vi "Status.Builder.New.vi"(8 "error in (no error)":errorcluster, 10 "Builder State Pointer":refnum<class "DSF.Engine.Pointer.Status.Builder.State.lvclass">, 11 "Builder Status type":refnum<class "Status.Builder.lvclass">) -> (0 "error out":errorcluster, 3 "Builder Status":refnum<class "Status.Builder.lvclass">)   [LabVIEW 2017, in "DSF.Engine.lvlib" / "Status.Builder.lvclass"]
uses:
  Status.Builder.lvclass
  Pointer/DSF.Engine.Pointer.Status.Builder.State.lvclass
  Status.Builder.lvclass/Status.Builder.ctl
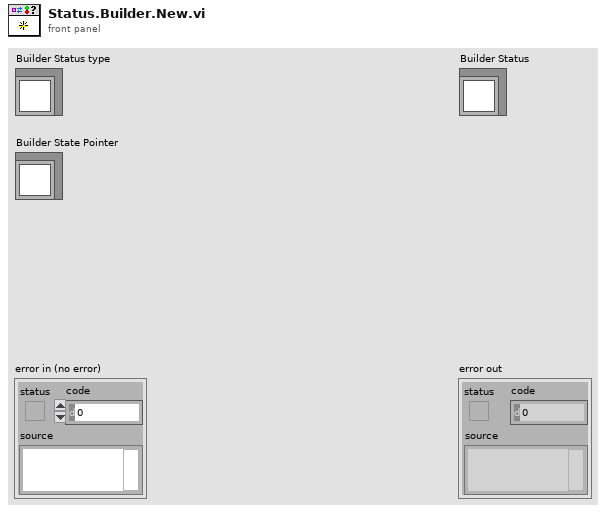
[diagram p1: front panel]
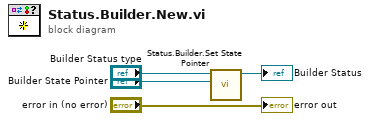
[diagram p0: block diagram]
diagram:
  n1 = call "Status.Builder.Set State Pointer.vi"("Builder State Pointer"="Builder State Pointer", "Builder Status in"="Builder Status type") -> ("Builder Status out"=→"Builder Status":refnum<class "Status.Builder.lvclass">)  [unwired: 9 in]
  "error out" <- "error in (no error)"
